vi "UHR-Fleezers Control (host) - 11.8.vi"() -> ()   [LabVIEW 2014] (continued)
                                tunnel: w980 -> [w981]
                                frame #0 {
                                n672 = property on="Trap Pos FB SP" class="DigNum (strict)"("Val(Sgnl)"=w981) -> ()  [unwired: 2 in, 2 out]
                                }
                                frame #1 {
                                n673 = Wait (ms)(milliseconds to wait=u32 700) -> ()  [unwired: 1 out]
                                }
                                frame #2 {
                                n674 = local read "Action (%)"() -> (w986:dbl)
                                n675 = Absolute Value(x=w986) -> (abs(x)=w985:dbl)
                                n676 = Greater?(x=w985, y=70.0) -> (0:w983:bool)
                                n677 = property on="Remove Action Offset" class="Bool (strict)"("Val(Sgnl)"=w983) -> ()  [unwired: 2 in, 2 out]
                                }
                                frame #3 {
                                n678 = for {
                                N: 4 -> [_]
                                n679 = flat-sequence {
                                frame #0 {
                                n680 = Wait (ms)(milliseconds to wait=u32 500) -> ()  [unwired: 1 out]
                                }
                                frame #1 {
                                n681 = local read "Action (%)"() -> (w992:dbl)
                                n682 = Absolute Value(x=w992) -> (abs(x)=w991:dbl)
                                n683 = Greater?(x=w991, y=70.0) -> (0:w989:bool)
                                n684 = property on="Remove Action Offset" class="Bool (strict)"("Val(Sgnl)"=w989) -> ()  [unwired: 2 in, 2 out]
                                }
                                }
                                }
                                }
                                frame #4 {
                                n685 = local read "Shift confocal"() -> (w996:bool)
                                n686 = local read "Mean"() -> (w999:dbl)
                                n687 = Greater?(x=w999, y=11.0) -> (0:w995:bool)
                                n688 = Not(x=w995) -> (.not. x?=w994:bool)
                                n689 = And(x=w994, y=w996) -> (x .and. y?=w993:bool)
                                n690 = And(x=w995, y=w996) -> (x .and. y?=w997:bool)
                                n691 = case shown="True" w997 {
                                frame False {
                                }
                                frame True {
                                n692 = local read "Confocal X 2 (V)"() -> (w1002:dbl)
                                n693 = local read "Confocal Y 2 (V)"() -> (w1003:dbl)
                                n694 = property on="AO2" class="Slide (strict)"("Val(Sgnl)"=w1002) -> ()  [unwired: 2 in, 2 out]
                                n695 = property on="AO1" class="Slide (strict)"("Val(Sgnl)"=w1003) -> ()  [unwired: 2 in, 2 out]
                                }
                                }
                                n696 = case shown="True" w993 {
                                frame False {
                                }
                                frame True {
                                n697 = local read "Confocal X 1 (V)"() -> (w1000:dbl)
                                n698 = local read "Confocal Y 1 (V)"() -> (w1001:dbl)
                                n699 = property on="AO1" class="Slide (strict)"("Val(Sgnl)"=w1001) -> ()  [unwired: 2 in, 2 out]
                                n700 = property on="AO2" class="Slide (strict)"("Val(Sgnl)"=w1000) -> ()  [unwired: 2 in, 2 out]
                                }
                                }
                                }
                                frame #5 {
                                n701 = Wait (ms)(milliseconds to wait=u32 1500) -> ()  [unwired: 1 out]
                                }
                                frame #6 {
                                n702 = property on="Remove Offset" class="Bool (strict)"("Val(Sgnl)"=TRUE ("Value (Signaling)")) -> ()  [unwired: 2 in, 2 out]
                                n703 = property on="Rem fb disp offset" class="Bool (strict)"("Val(Sgnl)"=TRUE ("Value (Signaling)")) -> ()  [unwired: 2 in, 2 out]
                                }
                                }
                                }
                                frame True {
                                n704 = flat-sequence {
                                tunnel: w1007 -> [w1008]
                                frame #0 {
                                n705 = property on="Trap D (MHz)" class="DigNum (strict)"("Val(Sgnl)"=w1008) -> ()  [unwired: 2 in, 2 out]
                                }
                                frame #1 {
                                n706 = Wait (ms)(milliseconds to wait=u32 500) -> ()  [unwired: 1 out]
                                }
                                frame #2 {
                                n707 = local read "Shift confocal"() -> (w1012:bool)
                                n708 = local read "Mean"() -> (w1010:dbl)
                                n709 = Greater?(x=w1010, y=11.0) -> (0:w1013:bool)
                                n710 = Not(x=w1013) -> (.not. x?=w1014:bool)
                                n711 = And(x=w1014, y=w1012) -> (x .and. y?=w1016:bool)
                                n712 = And(x=w1013, y=w1012) -> (x .and. y?=w1015:bool)
                                n713 = case shown="True" w1015 {
                                frame False {
                                }
                                frame True {
                                n714 = local read "Confocal Y 2 (V)"() -> (w1020:dbl)
                                n715 = local read "Confocal X 2 (V)"() -> (w1019:dbl)
                                n716 = property on="AO1" class="Slide (strict)"("Val(Sgnl)"=w1020) -> ()  [unwired: 2 in, 2 out]
                                n717 = property on="AO2" class="Slide (strict)"("Val(Sgnl)"=w1019) -> ()  [unwired: 2 in, 2 out]
                                }
                                }
                                n718 = case shown="True" w1016 {
                                frame False {
                                }
                                frame True {
                                n719 = local read "Confocal X 1 (V)"() -> (w1017:dbl)
                                n720 = local read "Confocal Y 1 (V)"() -> (w1018:dbl)
                                n721 = property on="AO2" class="Slide (strict)"("Val(Sgnl)"=w1017) -> ()  [unwired: 2 in, 2 out]
                                n722 = property on="AO1" class="Slide (strict)"("Val(Sgnl)"=w1018) -> ()  [unwired: 2 in, 2 out]
                                }
                                }
                                }
                                }
                                }
                                }
                                }
                              }
                            }
                            frame "Raster" {
                              n723 = property on="Trap Raster Scan" class="Bool (strict)"("Val(Sgnl)"=TRUE ("Value (Signaling)")) -> ()  [unwired: 2 in, 2 out]
                            }
                          }
                          n724 = local read "Time (s)"() -> (w953:dbl)
                          "Fl. High" <- TRUE ("Yanking")
                        }
                        frame #1 {
                          n725 = local read "Auto F Reset"() -> (w1022:bool)
                          n726 = case shown="True" w1022 {
                            tunnel: w1027 -> [_ w1031]
                            tunnel: w1026 -> [_ w1030]
                            tunnel: w1025 -> [_ w1029]
                            tunnel: w1023 -> [_ w1028]
                            frame False {
                            }
                            frame True {
                              n727 = node-c288() -> (w1033:T21)  [unwired: 4 out]
                              n728 = timed-loop {
                                timing: w1033 -> [_]
                                timing-out: [_] -> w1032
                                tunnel: w1031 -> [w1051]
                                tunnel: w1030 -> [w1050]
                                tunnel: w1029 -> [w1049]
                                tunnel: w1028 -> [w1048]
                                stop <- w1034 stop-if-true
                                n729 = node-c288() -> ()  [unwired: 2 out]
                                n730 = local read "Fl. D Thresh. (kHz)"() -> (w1042:dbl)
                                n731 = local read "Fl. Triggered..."() -> (w1047:bool)
                                n732 = local read "Delta Fl. 1"() -> (w1038:dbl)
                                n733 = local read "Delta Fl. 2"() -> (w1036:dbl)
                                n734 = local read "Stop All"() -> (w1045:bool)
                                n735 = local read "APD to Watch"() -> (w1037:bool)
                                n736 = Select(t=w1038, s=w1037, f=w1036) -> (s? t:f=w1035:dbl)
                                n737 = Not(x=w1047) -> (.not. x?=w1046:bool)
                                n738 = Multiply(x=w1042, y=1000.0) -> (x*y=w1041:dbl)
                                n739 = Negate(x=w1041) -> (-x=w1040:dbl)
                                n740 = Less?(x=w1035, y=w1040) -> (x < y?=w1044:bool)
                                n741 = Compound Arithmetic op=OR(w1044, w1045, w1046, "Reset Force") -> (w1034:bool)
                                n742 = case shown="True" w1034 {
                                tunnel: w1051 -> [_ w1066]
                                tunnel: w1050 -> [_ w1065]
                                tunnel: w1049 -> [_ w1055]
                                tunnel: w1048 -> [_ w1057]
                                frame False {
                                }
                                frame True {
                                n743 = local read "Time (s)"() -> (w1056:dbl)
                                n744 = case shown="\"Yank\"" w1065 {
                                tunnel: w1066 -> [_ w1069]
                                tunnel: w1057 -> [_ w1067]
                                frame "Image", Default {
                                }
                                frame "Yank" {
                                n745 = flat-sequence {
                                tunnel: [w1075] -> w1070
                                tunnel: w1069 -> [w1075]
                                tunnel: [w1071] -> w1068
                                tunnel: w1067 -> [w1071]
                                tunnel: w1070 -> [w1078]
                                tunnel: w1068 -> [w1076]
                                frame #0 {
                                n746 = local read "Yank Delay (s)"() -> (w1074:dbl)
                                n747 = Multiply(x=w1074, y=1000.0) -> (x*y=w1072:dbl)
                                n748 = Wait (ms)(milliseconds to wait=w1072) -> ()  [unwired: 1 out]
                                }
                                frame #1 {
                                n749 = local read "Yank to which?"() -> (w1077:bool)
                                n750 = case shown="False" w1077 {
                                tunnel: w1078 -> [_ w1106]
                                tunnel: w1076 -> [w1079 _]
                                frame False {
                                n751 = flat-sequence {
                                tunnel: w1079 -> [w1080]
                                frame #0 {
                                n752 = property on="Trap Pos FB SP" class="DigNum (strict)"("Val(Sgnl)"=w1080) -> ()  [unwired: 2 in, 2 out]
                                }
                                frame #1 {
                                n753 = Wait (ms)(milliseconds to wait=u32 700) -> ()  [unwired: 1 out]
                                }
                                frame #2 {
                                n754 = local read "Action (%)"() -> (w1085:dbl)
                                n755 = Absolute Value(x=w1085) -> (abs(x)=w1084:dbl)
                                n756 = Greater?(x=w1084, y=70.0) -> (0:w1082:bool)
                                n757 = property on="Remove Action Offset" class="Bool (strict)"("Val(Sgnl)"=w1082) -> ()  [unwired: 2 in, 2 out]
                                }
                                frame #3 {
                                n758 = for {
                                N: 4 -> [_]
                                n759 = flat-sequence {
                                frame #0 {
                                n760 = Wait (ms)(milliseconds to wait=u32 500) -> ()  [unwired: 1 out]
                                }
                                frame #1 {
                                n761 = local read "Action (%)"() -> (w1091:dbl)
                                n762 = Absolute Value(x=w1091) -> (abs(x)=w1090:dbl)
                                n763 = Greater?(x=w1090, y=70.0) -> (0:w1088:bool)
                                n764 = property on="Remove Action Offset" class="Bool (strict)"("Val(Sgnl)"=w1088) -> ()  [unwired: 2 in, 2 out]
                                }
                                }
                                }
                                }
                                frame #4 {
                                n765 = local read "Shift confocal"() -> (w1096:bool)
                                n766 = local read "Mean"() -> (w1098:dbl)
                                n767 = Greater?(x=w1098, y=11.0) -> (0:w1095:bool)
                                n768 = Not(x=w1095) -> (.not. x?=w1094:bool)
                                n769 = And(x=w1095, y=w1096) -> (x .and. y?=w1093:bool)
                                n770 = And(x=w1094, y=w1096) -> (x .and. y?=w1092:bool)
                                n771 = case shown="True" w1093 {
                                frame False {
                                }
                                frame True {
                                n772 = local read "Confocal Y 2 (V)"() -> (w1102:dbl)
                                n773 = local read "Confocal X 2 (V)"() -> (w1101:dbl)
                                n774 = property on="AO2" class="Slide (strict)"("Val(Sgnl)"=w1101) -> ()  [unwired: 2 in, 2 out]
                                n775 = property on="AO1" class="Slide (strict)"("Val(Sgnl)"=w1102) -> ()  [unwired: 2 in, 2 out]
                                }
                                }
                                n776 = case shown="True" w1092 {
                                frame False {
                                }
                                frame True {
                                n777 = local read "Confocal X 1 (V)"() -> (w1099:dbl)
                                n778 = local read "Confocal Y 1 (V)"() -> (w1100:dbl)
                                n779 = property on="AO1" class="Slide (strict)"("Val(Sgnl)"=w1100) -> ()  [unwired: 2 in, 2 out]
                                n780 = property on="AO2" class="Slide (strict)"("Val(Sgnl)"=w1099) -> ()  [unwired: 2 in, 2 out]
                                }
                                }
                                }
                                frame #5 {
                                n781 = Wait (ms)(milliseconds to wait=u32 1500) -> ()  [unwired: 1 out]
                                }
                                frame #6 {
                                n782 = property on="Rem fb disp offset" class="Bool (strict)"("Val(Sgnl)"=TRUE ("Value (Signaling)")) -> ()  [unwired: 2 in, 2 out]
                                n783 = property on="Remove Offset" class="Bool (strict)"("Val(Sgnl)"=TRUE ("Value (Signaling)")) -> ()  [unwired: 2 in, 2 out]
                                }
                                }
                                }
                                frame True {
                                n784 = flat-sequence {
                                tunnel: w1106 -> [w1107]
                                frame #0 {
                                n785 = property on="Trap D (MHz)" class="DigNum (strict)"("Val(Sgnl)"=w1107) -> ()  [unwired: 2 in, 2 out]
                                }
                                frame #1 {
                                n786 = Wait (ms)(milliseconds to wait=u32 500) -> ()  [unwired: 1 out]
                                }
                                frame #2 {
                                n787 = local read "Shift confocal"() -> (w1113:bool)
                                n788 = local read "Mean"() -> (w1115:dbl)
                                n789 = Greater?(x=w1115, y=11.0) -> (0:w1112:bool)
                                n790 = Not(x=w1112) -> (.not. x?=w1111:bool)
                                n791 = And(x=w1112, y=w1113) -> (x .and. y?=w1110:bool)
                                n792 = And(x=w1111, y=w1113) -> (x .and. y?=w1109:bool)
                                n793 = case shown="True" w1110 {
                                frame False {
                                }
                                frame True {
                                n794 = local read "Confocal Y 2 (V)"() -> (w1119:dbl)
                                n795 = local read "Confocal X 2 (V)"() -> (w1118:dbl)
                                n796 = property on="AO2" class="Slide (strict)"("Val(Sgnl)"=w1118) -> ()  [unwired: 2 in, 2 out]
                                n797 = property on="AO1" class="Slide (strict)"("Val(Sgnl)"=w1119) -> ()  [unwired: 2 in, 2 out]
                                }
                                }
                                n798 = case shown="True" w1109 {
                                frame False {
                                }
                                frame True {
                                n799 = local read "Confocal Y 1 (V)"() -> (w1117:dbl)
                                n800 = local read "Confocal X 1 (V)"() -> (w1116:dbl)
                                n801 = property on="AO2" class="Slide (strict)"("Val(Sgnl)"=w1116) -> ()  [unwired: 2 in, 2 out]
                                n802 = property on="AO1" class="Slide (strict)"("Val(Sgnl)"=w1117) -> ()  [unwired: 2 in, 2 out]
                                }
                                }
                                }
                                }
                                }
                                }
                                }
                                }
                                }
                                }
                                n803 = local read "Messages"() -> (w1064:string)
                                n804 = Subtract(x=w1056, y=w1055) -> (x-y=w1062:dbl)
                                "Duration (s)" <- w1062
                                n805 = Number To Decimal String(number=w1062, width (-)=i16 0) -> (decimal integer string=w1060:string)
                                n806 = Concatenate Strings(w1060, " s fluorescence event." ("string")) -> (w1058:string)
                                n807 = call "Update messages.vi"("Message to add"=w1058, "Old message string"=w1064) -> ("New message string"=w1063:string)
                                n808 = local write "Reset Force"(FALSE ("Reset Force")) -> ()
                                n809 = local write "Waiting"(TRUE ("Waiting")) -> ()
                                n810 = local write "Messages"(w1063) -> ()
                                n811 = local write "Fl. High"(FALSE ("Fl. High")) -> ()
                                n812 = call <vilib>:"Beep.vi"() -> ()  [unwired: 3 in, 9 out]
                                }
                                }
                                n813 = node-c288() -> ()  [unwired: 2 out]
                              }
                              n814 = node-c288(w1032) -> ()  [unwired: 1 out]
                            }
                          }
                        }
                      }
                      n815 = local read "Trap Pos FB SP"() -> (w940:fxp<+/-,16,1>)
                      n816 = local read "Trap D (MHz)"() -> (w945:dbl)
                    }
                  }
                }
                frame #1 {
                  n817 = local read "Stop All"() -> (w1129:bool)
                  n818 = local read "Fl. Triggered..."() -> (w1127:bool)
                  n819 = Not(x=w1127) -> (.not. x?=w1128:bool)
                  n820 = Or(x=w1128, y=w1129) -> (x .or. y?=w1126:bool)
                }
              }
              n821 = case shown="True" w715 {
                frame False {
                }
                frame True {
                  n822 = local read "Confocal Y 1 (V)"() -> (w725:dbl)
                  n823 = local read "Confocal X 1 (V)"() -> (w724:dbl)
                  n824 = property on="AO2" class="Slide (strict)"("Val(Sgnl)"=w724) -> ()  [unwired: 2 in, 2 out]
                  n825 = property on="AO1" class="Slide (strict)"("Val(Sgnl)"=w725) -> ()  [unwired: 2 in, 2 out]
                }
              }
              n826 = case shown="True" w715 {
                frame False {
                }
                frame True {
                  w723 = FALSE ("Fl. High")
                  n827 = local write "Waiting"(w723) -> ()
                  n828 = local write "Fl. High"(w723) -> ()
                }
              }
              n829 = node-c288() -> ()  [unwired: 2 out]
            }
            n830 = node-c288(w713) -> ()  [unwired: 1 out]
          }
        }
      }
      event "Stop All": Value Change {
        n831 = event-data() -> ()  [unwired: 7 out]
        n832 = local read "Stop All"() -> (w1134:bool)
      }
    }
    n833 = node-c288() -> ()  [unwired: 2 out]
  }
  n834 = property on="Saved trap pos" class="WFGraph (strict)"("Visible"=TRUE) -> ()  [unwired: 2 in, 2 out]
  n835 = property on="Trap Delta Graph" class="WFGraph (strict)"("Visible"=FALSE) -> ()  [unwired: 2 in, 2 out]
  n836 = local write "Trap pos"(TRUE ("Trap pos")) -> ()
  n837 = node-c288(2 ("Processor")) -> (w108:T21)  [unwired: 3 out]
  n838 = timed-loop "Control parameters (event loop)" {
    tunnel: w18 -> [w1143]
    shift-right: [w1142] -> _
    shift-left: errorcluster {"status"=FALSE, "code"=0, "source"=""} ("error out") -> [w1141]
    tunnel: [w1140] -> _
    timing: w108 -> [_]
    timing-out: [_] -> w107
    tunnel: w81 -> [w1139]
    tunnel: w22 -> [w1138]
    tunnel: w21 -> [w1137]
    tunnel: w20 -> [w1136]
    tunnel: w19 -> [w1135]
    stop <- w1140 stop-if-true
    n839 = node-c288() -> ()  [unwired: 2 out]
    n840 = event shown="[46] \"Sample Channel Flow\": Value Change" {
      selector: _ -> [_ _ _ _ _ _ _ _ _ _ _ _ _ _ _ _ _ _ _ _ _ _ _ _ _ _ _ _ _ _ _ _ _ _ _ _ _ _ _ _ _ _ _ _ _ _ _ _ _ _ _ _ _ _ _ _ _ _ _ _ _ _ _ _ _ _ _ _ _ _ _ _ _ _ _ _ _ _ _ _]
      dyn-events: _ -> [_ _ _ _ _ _ _ _ _ _ _ _ _ _ _ _ _ _ _ _ _ _ _ _ _ _ _ _ _ _ _ _ _ _ _ _ _ _ _ _ _ _ _ _ _ _ _ _ _ _ _ _ _ _ _ _ _ _ _ _ _ _ _ _ _ _ _ _ _ _ _ _ _ _ _ _ _ _ _ _]
      timeout: _ -> [_ _ _ _ _ _ _ _ _ _ _ _ _ _ _ _ _ _ _ _ _ _ _ _ _ _ _ _ _ _ _ _ _ _ _ _ _ _ _ _ _ _ _ _ _ _ _ _ _ _ _ _ _ _ _ _ _ _ _ _ _ _ _ _ _ _ _ _ _ _ _ _ _ _ _ _ _ _ _ _]
      tunnel: w1143 -> [w1181 _ _ _ w1219 _ w1241 _ _ _ _ w1307 _ _ w1350 w1356 w1361 w1367 w1403 w1421 w1428 _ w1440 w1444 w1455 w1466 w1477 w1488 w1499 w1510 w1537 w1631 w1638 w1676 _ _ w1736 w1740 w1751 w1755 w1759 _ w1767 _ _ _ _ _ _ _ _ _ _ _ _ _ _ _ _ _ w2148 _ w2165 _ w2172 w2190 _ w2197 w2205 w2220 w2231 w2237 _ w2246 _ w2265 _ _ _ w2340]
      tunnel: [w1180 _ _ _ w1209 _ w1240 _ _ w1272 _ w1286 _ _ w1349 w1352 w1358 w1364 w1402 w1419 w1427 _ w1438 _ w1449 w1460 w1471 w1482 w1493 w1504 w1535 w1629 w1636 w1674 _ _ w1734 w1738 w1741 w1753 w1757 _ w1765 _ _ _ _ _ _ _ _ _ _ _ _ _ _ _ _ _ w2146 _ _ _ _ w2187 _ _ _ _ _ _ _ _ _ _ _ _ _ w2338] -> w1142
      tunnel: w1141 -> [w1179 _ _ _ w1218 _ w1239 _ _ w1272 _ w1306 _ _ w1348 w1351 w1357 w1363 w1401 w1420 w1426 _ w1439 w1443 w1454 w1465 w1476 w1487 w1498 w1509 w1536 w1630 w1637 w1675 _ _ w1735 w1739 w1750 w1754 w1758 _ w1766 _ _ _ _ _ _ _ _ _ _ _ _ _ _ _ _ _ w2147 _ w2164 _ w2171 w2189 _ w2196 w2204 w2219 w2230 w2236 _ w2245 _ w2264 _ _ _ w2339]
      tunnel: [_ _ _ _ _ _ _ _ _ w1271 _ _ _ _ _ _ _ _ _ _ _ _ _ _ _ _ _ _ _ _ _ _ _ _ _ _ _ _ _ _ _ _ _ _ _ _ _ _ _ _ _ _ _ _ _ _ _ _ _ _ _ _ _ _ _ _ _ _ _ _ _ _ _ _ _ _ _ _ _ _] -> w1140
      tunnel: [_ _ _ _ _ _ _ "Round T1 X" _ _ _ _ _ _ _ _ _ _ _ _ _ _ _ _ _ _ _ _ _ _ _ _ _ _ _ _ _ _ _ _ _ _ _ _ _ _ _ _ _ _ _ _ _ _ _ _ _ _ _ _ _ _ _ _ _ _ _ _ _ _ _ _ _ _ _ _ _ _ _ _] -> _
      tunnel: [_ _ _ "Adjust Scale\nto Mean" _ _ _ _ _ _ _ _ _ _ _ _ _ _ _ _ _ _ "Test ttrig" _ _ _ _ _ _ _ _ _ _ _ _ _ _ _ _ _ _ _ _ _ _ _ _ _ _ _ "Flush Sample" "Flush Pump 3" "Flush Pump 1" "Clear Volume" _ _ _ _ _ _ _ _ _ _ _ _ _ _ _ _ _ _ _ _ _ _ _ _ _ _] -> _
      tunnel: [_ _ _ _ _ _ _ _ "Round T2 X" _ "Delayed Interlace Start" _ _ _ _ _ _ _ _ _ _ _ _ _ _ _ _ _ _ _ _ _ _ _ _ _ _ _ _ _ _ _ _ _ _ _ _ _ _ _ _ _ _ _ _ _ _ _ _ _ _ _ _ _ _ _ _ _ _ _ _ _ _ _ _ _ _ _ _ _] -> _
      tunnel: w1139 -> [_ _ _ _ _ _ _ _ _ _ _ _ _ _ _ _ _ _ _ _ _ _ _ _ _ _ _ _ _ _ _ _ _ _ _ _ _ _ _ _ _ _ _ _ _ _ w1925 w1943 w1950 w1955 w1961 _ _ w2060 _ _ _ _ _ _ _ _ _ _ _ _ _ _ _ _ _ _ _ _ _ _ _ _ _ _]
      tunnel: w1138 -> [_ _ _ _ _ _ _ _ _ _ _ _ _ _ _ _ _ _ _ _ _ _ _ _ _ _ _ _ _ _ _ _ _ _ _ _ _ _ _ _ _ _ _ _ w1841 _ _ _ _ _ _ w1991 _ _ w2067 _ w2076 _ w2090 _ _ _ _ _ _ _ _ _ _ _ _ _ _ _ _ _ _ _ _ _]
      tunnel: w1137 -> [_ _ _ _ _ _ _ _ _ _ _ _ _ _ _ _ _ _ _ _ _ _ _ _ _ _ _ _ _ _ _ _ _ _ _ _ _ _ _ _ _ _ _ _ _ _ _ _ _ _ _ _ _ _ _ _ _ _ _ _ _ _ _ _ _ _ _ _ _ _ _ _ _ _ _ _ _ _ _ _]
      tunnel: w1136 -> [_ _ _ _ _ _ _ _ _ _ _ _ _ _ _ _ _ _ _ _ _ _ _ _ _ _ _ _ _ _ _ _ _ _ _ _ _ _ _ _ _ _ _ w1778 _ _ _ _ _ _ _ _ w2021 _ _ w2072 _ w2083 _ w2115 _ _ _ _ _ _ _ _ _ _ _ _ _ _ _ _ _ _ _ _]
      tunnel: w1135 -> [_ _ _ _ _ _ _ _ _ _ _ _ _ _ _ _ _ _ _ _ _ _ _ _ _ _ _ _ _ _ _ _ _ _ _ _ _ _ _ _ _ _ _ _ _ _ _ _ _ _ _ _ _ _ _ _ _ _ _ _ _ _ _ _ _ _ _ _ _ _ _ _ _ _ _ _ _ _ _ _]
      event "AI Count (ticks)", "Sets to FIFO (Traps)", "Save ave N", "FPGA Ave.", "# Samples/channel", "N sets to save": Value Change {
        # "So that if 'Save ave N' is updated, the AOD scanning code updates too."
        n841 = event-data() -> ()  [unwired: 6 out]
        n842 = local read "AI Count (ticks)"() -> (w1161:u32)
        n843 = Boolean To (0,1)(Boolean="Sets to FIFO (Traps)") -> (0, 1=w1171:cluster{"Set 1":i16, "Set 2":i16, "Set 3":i16})
        n844 = Cluster To Array(cluster=w1171) -> (array=w1170:i16[])
        n845 = xnode "Read/Write Control"("FPGA VI Reference In"=w1181, "error in"=w1179, "ai count"=w1161, "AI1 Sets to FIFO"="Sets to FIFO (Traps)", "N of AI1 Int Acq Sets"="N Acq Sets (Traps + Fl.)") -> ("error out"=w1180:errorcluster)  [unwired: 1 out]
        n846 = To Unsigned Long Integer(number=w1170) -> (unsigned 32bit integer=w1150:u32[])
        n847 = local read "Scan steps (AOD)"() -> (w1172:u64)
        n848 = Multiply(x=w1161, y="N Acq Sets (Traps + Fl.)") -> (x*y=w1159:u32)
        n849 = Divide(x=40000000.0, y=w1161) -> (x/y=w1153:dbl)
        "AI rate (Hz)" <- w1153
        "Ave. Rate (Hz)" <- w1153
        n850 = Add Array Elements(numeric array=w1150) -> (sum=w1162:u32)
        "Trap Sets" <- w1162
        n851 = Reciprocal(x=w1153) -> (1/x=→"Ave. Period (s)":dbl)
        n852 = property on="Scan steps (AOD)" class="DigNum (strict)"("Val(Sgnl)"=w1172) -> ()  [unwired: 2 in, 2 out]
        n853 = Divide(x=w1153, y="N Acq Sets (Traps + Fl.)") -> (x/y=w1176:dbl)
        "Data Rate (Hz)" <- w1176
        n854 = Reciprocal(x=w1176) -> (1/x=→"Data Period (s)":dbl)
        n855 = local read "Save ave N"() -> (w1175:dbl)
        n856 = Divide(x=w1176, y=w1175) -> (x/y=w1174:dbl)
        "Save Data Rate (Hz)" <- w1174
        n857 = Reciprocal(x=w1174) -> (1/x=→"Save Data Period (s)":dbl)
        n858 = Multiply(x=w1159, y="# Samples/trap") -> (x*y=w1157:u32)
        "Counts/DMA" <- w1157
        n859 = property on="Trap Disp. Downsample" class="DigNum (strict)"("Maximum"="# Samples/trap") -> ()  [unwired: 2 in, 2 out]
        n860 = Multiply(x=w1162, y="# Samples/trap") -> (x*y=w1151:u32)
        "# Samples/channel" <- w1151
        n861 = Multiply(x=w1151, y=u32 8) -> (x*y=→"Trap AI Elements/DMA read":u32)
        n862 = local read "APD Int. Count"() -> (w1158:u32)
        n863 = Multiply(x=w1151, y=u32 3) -> (x*y=→"Trap Pos Elements/DMA read":u32)
        n864 = Divide(x=w1157, y=w1158) -> (x/y=w1148:dbl)
        "APD Samples/FIFO Acq." <- w1148
        n865 = Divide(x=w1157, y=40000000.0) -> (x/y=w1155:dbl)
        "DMA Update Period (s)" <- w1155
        n866 = Multiply(x=2.0, y=w1148) -> (x*y=→"APD Elements/DMA read":dbl)
        n867 = property on="APD Disp. Downsample" class="DigNum (strict)"("Maximum"=w1148) -> ()  [unwired: 2 in, 2 out]
        n868 = local read "N sets to save"() -> (w1168:u32)
        n869 = Multiply(x=w1155, y=w1168) -> (x*y=→"Total Time (s)":dbl)
        "FPGA Averaging" <- FALSE ("FPGA Averaging")
      }
      event "Remove Offset": Value Change {
        n870 = event-data() -> ()  [unwired: 7 out]
        n871 = local write "Remove Offset"(FALSE ("Remove Offset")) -> ()
        n872 = local read "Bead Mean (nm)"() -> (w1183:dbl)
        n873 = local read "Offset (nm)"() -> (w1184:dbl)
        n874 = Add(x=w1183, y=w1184) -> (x+y=w1182:dbl)
        n875 = local write "Offset (nm)"(w1182) -> ()
        n876 = disable-structure shown="Disabled" {
          frame Disabled {
            n877 = local read "Bead Mean (nm)"() -> (w1189:dbl)
            n878 = Add(y=w1189) -> (x=w1188:dbl, x+y=w1187:dbl)
            n879 = Subtract(x=w1189, y=w1188) -> (x-y=w1186:dbl)
            n880 = property on="Bead Separation" class="WFChart (strict)"("YScale.Minimum"=w1186) -> ()  [unwired: 2 in, 2 out]
            n881 = property on="Bead Separation" class="WFChart (strict)"("YScale.Maximum"=w1187) -> ()  [unwired: 2 in, 2 out]
          }
          frame Enabled {
          }
        }
      }
      event "Detector Type": Value Change {
        n882 = event-data() -> ()  [unwired: 7 out]
        n883 = local read "AI labels"() -> (w1190:string[])
        n884 = property on="High Res. Display" class="Ring (strict)"("Strings []"=w1190) -> ()  [unwired: 2 in, 2 out]
        n885 = Build Array (concatenate)(w1190, "none") -> (w1191:string[])
        n886 = property on="FFT 1 Choice 1" class="Ring (strict)"("Strings []"=w1191) -> ()  [unwired: 2 in, 2 out]
        n887 = property on="FFT 1 Choice 2" class="Ring (strict)"("Strings []"=w1191) -> ()  [unwired: 2 in, 2 out]
        n888 = property on="FFT 2 Choice 1" class="Ring (strict)"("Strings []"=w1191) -> ()  [unwired: 2 in, 2 out]
        n889 = property on="FFT 2 Choice 2" class="Ring (strict)"("Strings []"=w1191) -> ()  [unwired: 2 in, 2 out]
        n890 = Bundle("APD 1", "APD 2") -> (w1194:cluster{string, string})  [unwired: 1 out]
        n891 = Cluster To Array(cluster=w1194) -> (array=w1192:string[])
        n892 = Build Array (concatenate)(w1192, w1191) -> (w1196:string[])
        n893 = Array Size(array=w1196) -> (size(s)=w1197:i32)
        n894 = property on="Signals to Plot" class="LstBox (strict)"("Item Names"=w1196) -> ()  [unwired: 2 in, 2 out]
        n895 = property on="Signals to Plot" class="LstBox (strict)"("Number of Rows"=w1197) -> ()  [unwired: 2 in, 2 out]
        n896 = property on="All Signals" class="WFChart (strict)"("LegNumRows"=w1197) -> ()  [unwired: 2 in, 2 out]
      }
      event "Adjust Scale\nto Mean": Value Change {
        n897 = event-data() -> ()  [unwired: 7 out]
        n898 = local read "APD 1 Rate (Hz)"() -> (w1206:dbl)
        n899 = Multiply(x=1000.0, y="Above (kHz)") -> (x*y=w1204:dbl)
        n900 = Multiply(x=1000.0, y="Below (kHz)") -> (x*y=w1202:dbl)
        n901 = Add(x=w1204, y=w1206) -> (x+y=w1199:dbl)
        n902 = Subtract(x=w1206, y=w1202) -> (x-y=w1200:dbl)
        n903 = property on="APD Chart" class="WFChart (strict)"("YScale.Minimum"=w1200) -> ()  [unwired: 2 in, 2 out]
        n904 = property on="APD Chart" class="WFChart (strict)"("YScale.Maximum"=w1199) -> ()  [unwired: 2 in, 2 out]
      }
      event "Phase adj. (AI1)", "+ phase (AI1)", "- phase (AI1)": Value Change {
        n905 = event-data() -> ()  [unwired: 7 out]
        n906 = Negate(x="Phase adj. (AI1)") -> (-x=w1216:i16)
        n907 = Select(t=w1216, s="- phase (AI1)", f="Phase adj. (AI1)") -> (s? t:f=w1215:i16)
        n908 = xnode "Read/Write Control"("FPGA VI Reference In"=w1219, "error in"=w1218, "Phase count adjustment"=w1215) -> ("FPGA VI Reference Out"=w1214:T19, "error out"=w1213:errorcluster)
        n909 = Or(x="- phase (AI1)", y="+ phase (AI1)") -> (x .or. y?=w1210:bool)
        n910 = xnode "Read/Write Control"("FPGA VI Reference In"=w1214, "error in"=w1213, "+ phase"=w1210) -> ("error out"=w1209:errorcluster)  [unwired: 1 out]
      }
      event "Signals to Plot": Double Click {
        w1222 = u32 9868950 ("Color Box")
        n911 = event-data() -> ("Row"=w1224:i32)  [unwired: 9 out]
        n912 = property on="All Signals" class="WFChart (strict)"("Active Plot"=w1224) -> (error out=w1235:errorcluster)  [unwired: 2 in, 1 out]
        n913 = property on="All Signals" class="WFChart (strict)" props=["Plot", "Visible?", "Plot", "Plot Color"](error in=w1235) -> (error out=w1234:errorcluster, "Plot.Visible?"=w1233:bool)  [unwired: 1 in, 2 out]
        n914 = Select(t=FALSE ("Plot.Visible"), s=w1233, f=TRUE ("Plot.Visible")) -> (s? t:f=w1228:bool)
        n915 = property on="All Signals" class="WFChart (strict)"(error in=w1234, "Plot.Visible?"=w1228) -> (error out=w1230:errorcluster)  [unwired: 1 in, 1 out]
        n916 = property on="All Signals" class="WFChart (strict)"(error in=w1230) -> (error out=w1225:errorcluster, "Plot.Plot Color"=w1229:u32)  [unwired: 1 in, 1 out]
        n917 = property on="Signals to Plot" class="LstBox (strict)"(error in=w1225, "Active Row"=w1224) -> (error out=w1223:errorcluster)  [unwired: 1 in, 1 out]
        n918 = Select(t=w1229, s=w1228, f=u32 0) -> (s? t:f=w1226:u32)
        n919 = property on="Signals to Plot" class="LstBox (strict)"(error in=w1223, "CellFontColor"=w1226, "SelColor"=w1222, "CellBG"=w1222, "CellFontSize"=u32 20 ("Active Row:Cell Font:Size"), "CellFontBold"=TRUE ("Active Row:Cell Font:Bold")) -> ()  [unwired: 1 in, 2 out]
      }
      event "BD 1 Frequency 1 (MHz)", "BD 1 Frequency 2 (MHz)", "BD 1 Frequency 3 (MHz)", "BD 2 Frequency 1 (MHz)", "BD 2 Frequency 2 (MHz)", "BD 2 Frequency 3 (MHz)", "Trap D (MHz)": Value Change {
        n920 = event-data() -> ("CtlRef"=w1238:refnum<vi>)  [unwired: 6 out]
        n921 = control-ref of="Trap D (MHz)"() -> (w1237:refnum<vi>)
        n922 = Equal?(x=w1237, y=w1238) -> (x = y?=w1236:bool)
        n923 = case shown="False" "Oscillate Set 1" {
          tunnel: w1241 -> [w1261 _]
          tunnel: [w1260 w1264] -> w1240
          tunnel: w1239 -> [w1259 w1264]
          tunnel: w1236 -> [w1244 _]
          frame False {
            n924 = local read "BD 1 Frequency 2 (MHz)"() -> (w1248:dbl)
            n925 = local read "BD 1 Frequency 1 (MHz)"() -> (w1246:dbl)
            n926 = Subtract(x=w1248, y="Trap D (MHz)") -> (x-y=w1245:dbl)
            n927 = Select(t=w1245, s=w1244, f=w1246) -> (s? t:f=w1243:dbl)
            n928 = local read "Y RF Frequency Limits (MHz)"() -> (w1249:T16)
            n929 = local read "X RF Frequency Limits (MHz)"() -> (w1250:T16)
            n930 = local read "BD 1 Frequency 3 (MHz)"() -> (w1262:dbl)
            n931 = local write "BD 1 Frequency 1 (MHz)"(w1243) -> ()
            n932 = local read "BD 2 Frequency 1 (MHz)"() -> (w1253:dbl)
            n933 = local read "BD 2 Frequency 2 (MHz)"() -> (w1252:dbl)
            n934 = local read "BD 2 Frequency 3 (MHz)"() -> (w1263:dbl)
            n935 = call "set RF board frequency - interlace.vi"("Board 2 Frequency Limits"=w1249, "Board 1 Frequency Limits"=w1250, "error in"=w1259, "FPGA VI Reference In"=w1261, "Board 2 Frequency 3 (MHz)"=w1263, "Board 1 Frequency 3 (MHz)"=w1262, "Board 2 Frequency 2 (MHz)"=w1252, "Board 2 Frequency 1 (MHz)"=w1253, "Board 1 Frequency 2 (MHz)"=w1248, "Board 1 Frequency 1  (MHz)"=w1243) -> ("error out"=w1260:errorcluster)  [unwired: 1 out]
            n936 = Subtract(x=w1253, y=w1252) -> (x-y=w1257:dbl)
            n937 = Subtract(x=w1243, y=w1248) -> (x-y=w1258:dbl)
            n938 = Square(x=w1257) -> (x^2=w1255:dbl)
            n939 = Square(x=w1258) -> (x^2=w1256:dbl)
            n940 = Add(x=w1256, y=w1255) -> (x+y=w1254:dbl)
            n941 = Square Root(x=w1254) -> (sqrt(x)=w1251:dbl)
            n942 = local write "Trap D (MHz)"(w1251) -> ()
            n943 = property on="Initial D (MHz)" class="DigNum (strict)"("Val(Sgnl)"=w1251) -> ()  [unwired: 2 in, 2 out]
          }
          frame True {
          }
        }
      }
      event "Round T1 X": Value Change {
        n944 = event-data() -> ()  [unwired: 7 out]
        n945 = local read "BD 1 Frequency 1 (MHz)"() -> (w1267:dbl)
        n946 = Round To Nearest(number=w1267) -> (nearest integer value=w1266:dbl)
        n947 = property on="BD 1 Frequency 1 (MHz)" class="DigNum (strict)"("Val(Sgnl)"=w1266) -> ()  [unwired: 2 in, 2 out]
      }
      event "Round T2 X": Value Change {
        n948 = event-data() -> ()  [unwired: 7 out]
        n949 = local read "BD 1 Frequency 2 (MHz)"() -> (w1269:dbl)
        n950 = Round To Nearest(number=w1269) -> (nearest integer value=w1268:dbl)
        n951 = property on="BD 1 Frequency 2 (MHz)" class="DigNum (strict)"("Val(Sgnl)"=w1268) -> ()  [unwired: 2 in, 2 out]
      }
      event "Stop All": Value Change {
        n952 = event-data() -> ()  [unwired: 7 out]
        n953 = local read "Stop All"() -> (w1271:bool)
      }
      event "Delayed Interlace Start": Value Change {
        n954 = event-data() -> ()  [unwired: 7 out]
        n955 = flat-sequence {
          frame #0 {
            n956 = Multiply(x="Delay to Interlace (s)", y=1000.0) -> (x*y=w1274:dbl)
            n957 = Wait (ms)(milliseconds to wait=w1274) -> ()  [unwired: 1 out]
          }
          frame #1 {
            n958 = property on="Green laser mode" class="RadioBtnsControl (strict)"("Val(Sgnl)"=enum32{"Laser ON", "Laser OFF", "Interlace"}."Interlace" ("Value (Signaling)")) -> ()  [unwired: 2 in, 2 out]
          }
        }
      }
      event "BD 1 Amplitude 1 (%)", "BD 1 Amplitude 2 (%)", "BD 1 Amplitude 3 (%)", "BD 2 Amplitude 1 (%)", "BD 2 Amplitude 2 (%)", "BD 2 Amplitude 3 (%)", "Trap 1 ON", "Trap 2 ON", "Trap 3 ON", "Feedback On/Off", "All FB On/Off": Value Change {
        w1298 = i16 1 ("f")
        n959 = event-data() -> ()  [unwired: 7 out]
        n960 = local write "Trap 1 (ON/OFF)"("Trap 1 ON") -> ()
        n961 = local write "Trap 2 (ON/OFF)"("Trap 2 ON") -> ()
        n962 = Boolean To (0,1)(Boolean="Trap 3 ON") -> (0, 1=w1299:i16)
        n963 = Boolean To (0,1)(Boolean="Trap 1 ON") -> (0, 1=w1300:i16)
        n964 = Boolean To (0,1)(Boolean="Trap 2 ON") -> (0, 1=w1301:i16)
        n965 = Select(t=w1301, s="Trap ON/OFF X or Y Amp?", f=w1298) -> (s? t:f=w1296:i16)
        n966 = Select(t=w1300, s="Trap ON/OFF X or Y Amp?", f=w1298) -> (s? t:f=w1297:i16)
        n967 = Select(t=w1299, s="Trap ON/OFF X or Y Amp?", f=w1298) -> (s? t:f=w1295:i16)
        n968 = Select(t=w1298, s="Trap ON/OFF X or Y Amp?", f=w1301) -> (s? t:f=w1293:i16)
        n969 = Select(t=w1298, s="Trap ON/OFF X or Y Amp?", f=w1300) -> (s? t:f=w1294:i16)
        n970 = Select(t=w1298, s="Trap ON/OFF X or Y Amp?", f=w1299) -> (s? t:f=w1292:i16)
        n971 = And(x="All FB On/Off", y="Feedback On/Off") -> (x .and. y?=w1290:cluster{"Set 1":bool, "Set 2":bool})
        n972 = local read "BD 1 Amplitude 1 (%)"() -> (w1310:dbl)
        n973 = local read "BD 1 Amplitude 2 (%)"() -> (w1309:dbl)
        n974 = local read "BD 1 Amplitude 3 (%)"() -> (w1308:dbl)
        n975 = Unbundle By Name(w1290) -> ("Set 1"=w1285:bool, "Set 2"=w1282:bool)
        n976 = local read "Y RF Amplitude Limits (%)"() -> (w1278:T16)
        n977 = local read "X RF Amplitude Limits (%)"() -> (w1279:T16)
        n978 = local read "BD 2 Amplitude 1 (%)"() -> (w1311:dbl)
        n979 = local read "BD 2 Amplitude 2 (%)"() -> (w1312:dbl)
        n980 = local read "BD 2 Amplitude 3 (%)"() -> (w1313:dbl)
        n981 = And(x="Trap 2 ON", y=w1282) -> (x .and. y?=w1280:bool)
        n982 = And(x="Trap 1 ON", y=w1285) -> (x .and. y?=w1283:bool)
        n983 = Multiply(x=w1297, y=w1310) -> (x*y=w1305:dbl)
        n984 = Multiply(x=w1309, y=w1296) -> (x*y=w1303:dbl)
        n985 = Multiply(x=w1308, y=w1295) -> (x*y=w1304:dbl)
        n986 = Multiply(x=w1311, y=w1294) -> (x*y=w1314:dbl)
        n987 = Multiply(x=w1312, y=w1293) -> (x*y=w1315:dbl)
        n988 = Multiply(x=w1313, y=w1292) -> (x*y=w1316:dbl)
        n989 = call "set RF board amplitude - interlace.vi"("Board 2 Amplitude Limits"=w1278, "Board 1 Amplitude Limits"=w1279, "error in"=w1306, "FPGA VI Reference In"=w1307, "Board 2 Amplitude 3 (%)"=w1316, "Board 1 Amplitude 3 (%)"=w1304, "Board 2 Amplitude 2 (%)"=w1315, "Board 2 Amplitude 1 (%)"=w1314, "Board 1 Amplitude 2 (%)"=w1303, "Board 1 Amplitude 1 (%)"=w1305) -> ("error out"=w1287:errorcluster, "FPGA VI Reference Out"=w1288:T19)
        n990 = xnode "Read/Write Control"("FPGA VI Reference In"=w1288, "error in"=w1287, "FB On/Off Set 1"=w1283, "FB On/Off Set 2"=w1280) -> ("error out"=w1286:errorcluster)  [unwired: 1 out]
      }
      event "Load parameters": Value Change {
        n991 = event-data() -> ()  [unwired: 7 out]
        n992 = property on="Saved AOD Raster Scan Parameter Sets" class="Arr (strict)"() -> ("Index Values"=w1327:u32[])  [unwired: 2 in, 2 out]
        n993 = Index Array(array=w1327, index=0) -> (element=w1324:u32)
        n994 = local write "Load parameters"(FALSE ("Load parameters")) -> ()
        n995 = Index Array(array="Saved AOD Raster Scan Parameter Sets", index=w1324) -> (element=w1323:T26)
        n996 = Unbundle By Name(w1323) -> ("Scan Range AOD (nm) 2"=w1322:dbl, "Step Size AOD (nm) 2"=w1321:dbl, "Scan Speed AOD (nm/s) 2"=w1320:dbl, "Number of scans (AOD) 2"=w1319:u16)
        n997 = flat-sequence {
          tunnel: w1322 -> [w1330]
          tunnel: w1321 -> [w1329]
          tunnel: w1320 -> [w1328]
          tunnel: w1319 -> [w1331]
          frame #0 {
            n998 = local write "Scan Speed (nm/s)"(w1328) -> ()
            n999 = local write "Scan Range (nm)"(w1330) -> ()
            n1000 = local write "Step Size (nm)"(w1329) -> ()
          }
          frame #1 {
            n1001 = property on="Number of F/B Scans (AOD)" class="DigNum (strict)"("Val(Sgnl)"=w1331) -> ()  [unwired: 2 in, 2 out]
          }
        }
      }
      event "Trap 1 (ON/OFF)", "Trap 2 (ON/OFF)": Value Change {
        n1002 = event-data() -> ()  [unwired: 7 out]
        n1003 = property on="Trap 2 ON" class="Bool (strict)"("Val(Sgnl)"="Trap 2 (ON/OFF)") -> ()  [unwired: 2 in, 2 out]
        n1004 = property on="Trap 1 ON" class="Bool (strict)"("Val(Sgnl)"="Trap 1 (ON/OFF)") -> ()  [unwired: 2 in, 2 out]
      }
      event "DIO count 1 (ticks)", "DIO count 2 (ticks)", "DIO count 3 (ticks)", "Interlace", "Number Interlace Sets", "Not-Interlacing Set": Value Change {
        n1005 = event-data() -> ()  [unwired: 7 out]
        n1006 = local read "DIO count 3 (ticks)"() -> (w1344:u32)
        n1007 = local read "DIO count 1 (ticks)"() -> (w1346:u32)
        n1008 = local read "DIO count 2 (ticks)"() -> (w1345:u32)
        n1009 = To Unsigned Byte Integer(number="Not-Interlacing Set") -> (unsigned 8bit integer=w1335:u8)
        n1010 = Add(x=w1335, y=u8 1) -> (x+y=w1339:u8)
        n1011 = xnode "Read/Write Control"("FPGA VI Reference In"=w1350, "error in"=w1348, "DIO count 1 (ticks)"=w1346, "DIO count 2 (ticks)"=w1345, "DIO count 3 (ticks)"=w1344, "Interlace ON/OFF"="Interlace", "Number Interlace Cycles"="Number Interlace Sets", "Interlace Off Parameters"=w1339) -> ("error out"=w1349:errorcluster)  [unwired: 1 out]
        n1012 = Build Array(w1346, w1345, w1344) -> (w1337:u32[])
        n1013 = Split 1D Array(array=w1337, index="Number Interlace Sets") -> (first subarray=w1347:u32[])  [unwired: 1 out]
        n1014 = Index Array(array=w1337, index=w1335) -> (element=w1336:u32)
        n1015 = Add Array Elements(numeric array=w1347) -> (sum=w1341:u32)
        n1016 = Select(t=w1341, s="Interlace", f=w1336) -> (s? t:f=→"Total Counts (ticks)":u32)
      }
      event "Reset Feedback": Value Change {
        n1017 = event-data() -> ()  [unwired: 7 out]
        n1018 = Unbundle By Name("Reset Feedback") -> ("Set 1"=w1354:bool, "Set 2"=w1353:bool)
        n1019 = xnode "Read/Write Control"("FPGA VI Reference In"=w1356, "error in"=w1351, "FB Reset Set 1"=w1354, "FB Reset Set 2"=w1353) -> ("error out"=w1352:errorcluster)  [unwired: 1 out]
      }
      event "PID Gains": Value Change {
        n1020 = event-data() -> ()  [unwired: 7 out]
        n1021 = Unbundle By Name("PID Gains") -> ("Set 1"=w1360:T14, "Set 2"=w1359:T14)
        n1022 = xnode "Read/Write Control"("FPGA VI Reference In"=w1361, "error in"=w1357, "FB Gains Set 1"=w1360, "FB Gains Set 2"=w1359) -> ("error out"=w1358:errorcluster)  [unwired: 1 out]
      }
      event "AI2 to Setpoint", "Setpoints (V)": Value Change {
        n1023 = event-data() -> ()  [unwired: 7 out]
        n1024 = xnode "Read/Write Control"("FPGA VI Reference In"=w1367, "error in"=w1363) -> ("FPGA VI Reference Out"=w1366:T19, "error out"=w1365:errorcluster, "AI2 Y Sum Set 1"=w1374:i16, "AI2 Y Sum Set 2"=w1373:i16)
        n1025 = Cluster To Array(cluster="AI2 to Setpoint") -> (array=w1377:bool[])
        n1026 = local read "AI2 (V)"() -> (w1375:cluster{"Set 1":dbl, "Set 2":dbl})
        n1027 = Or Array Elements(Boolean array=w1377) -> (logical OR=w1378:bool)
        n1028 = Bundle By Name(cluster=w1375, "Set 1"=w1374, "Set 2"=w1373) -> (w1372:cluster{"Set 1":dbl, "Set 2":dbl})
        n1029 = Divide(x=w1372, y=3276.7) -> (x/y=w1371:cluster{"Set 1":dbl, "Set 2":dbl})
        "AI2 (V)" <- w1371
        n1030 = case shown="True" w1378 {
          tunnel: [w1381 w1398] -> w1370
          tunnel: "AI2 to Setpoint" -> [_ w1394]
          tunnel: "Setpoints (V)" -> [w1382 w1397]
          tunnel: w1371 -> [_ w1391]
          frame False {
            n1031 = Multiply(x=3276.7, y=w1382) -> (x*y=w1383:cluster{"Set 1":dbl, "Set 2":dbl})
            n1032 = To Word Integer(number=w1383) -> (16bit integer=w1381:cluster{"Set 1":i16, "Set 2":i16})
          }
          frame True {
            n1033 = Unbundle By Name(w1391) -> ("Set 1"=w1390:dbl, "Set 2"=w1389:dbl)
            n1034 = Unbundle By Name(w1397) -> ("Set 1"=w1396:dbl, "Set 2"=w1395:dbl)
            n1035 = Unbundle By Name(w1394) -> ("Set 1"=w1393:bool, "Set 2"=w1392:bool)
            n1036 = Select(t=w1390, s=w1393, f=w1396) -> (s? t:f=w1388:dbl)
            n1037 = Select(t=w1389, s=w1392, f=w1395) -> (s? t:f=w1387:dbl)
            n1038 = Bundle By Name(cluster=w1397, "Set 1"=w1388, "Set 2"=w1387) -> (w1385:cluster{"Set 1":dbl, "Set 2":dbl})
            n1039 = local write "Setpoints (V)"(w1385) -> ()
            n1040 = Multiply(x=3276.7, y=w1385) -> (x*y=w1386:cluster{"Set 1":dbl, "Set 2":dbl})
            n1041 = To Word Integer(number=w1386) -> (16bit integer=w1398:cluster{"Set 1":i16, "Set 2":i16})
          }
        }
        n1042 = Unbundle By Name(w1370) -> ("Set 1"=w1369:i16, "Set 2"=w1368:i16)
        n1043 = xnode "Read/Write Control"("FPGA VI Reference In"=w1366, "error in"=w1365, "FB Setpoint Set 1"=w1369, "FB Setpoint Set 2"=w1368) -> ("error out"=w1364:errorcluster)  [unwired: 1 out]
      }
      event "Invert GI": Value Change {
        n1044 = event-data() -> ()  [unwired: 7 out]
        n1045 = xnode "Read/Write Control"("FPGA VI Reference In"=w1403, "error in"=w1401, "Invert GI"="Invert GI", "Invert GI 2"="Invert GI") -> ("error out"=w1402:errorcluster)  [unwired: 1 out]
      }
      event "Green FB Setpoint (mV)", "Green FB Gains", "Green FB On/Off", "Current When FB OFF (%)", "Green int current ON count adj": Value Change {
        n1046 = event-data() -> ()  [unwired: 7 out]
        n1047 = local read "Green FB Setpoint (mV)"() -> (w1410:dbl)
        n1048 = local read "Current When FB OFF (%)"() -> (w1413:dbl)
        n1049 = Multiply(x=w1410, y=3.2767) -> (x*y=w1409:dbl)
        n1050 = Multiply(x=w1413, y=655.35) -> (x*y=w1414:dbl)
        n1051 = To Unsigned Word Integer(number=w1414) -> (unsigned 16bit integer=w1412:u16)
        n1052 = local read "Green int current ON count adj"() -> (w1417:u32)
        n1053 = local read "Green FB Gains"() -> (w1416:T14)
        n1054 = local read "Green Laser ON/Interlacing"() -> (w1407:bool)
        n1055 = local read "Green laser mode"() -> (w1406:enum32{"Laser ON", "Laser OFF", "Interlace"})
        n1056 = local read "Green FB On/Off"() -> (w1418:bool)
        n1057 = Equal?(x=w1406, y=enum32{"Laser ON", "Laser OFF", "Interlace"}."Interlace") -> (x = y?=w1404:bool)
        n1058 = Compound Arithmetic op=AND(w1404, w1418, w1407) -> (w1408:bool)
        n1059 = xnode "Read/Write Control"("FPGA VI Reference In"=w1421, "error in"=w1420, "Green FB Setpoint"=w1409, "Green FB On/Off"=w1408, "Current Out"=w1412, "Green int current ON count adj"=w1417, "Green FB Gains"=w1416) -> ("error out"=w1419:errorcluster)  [unwired: 1 out]
      }
      event "Green laser mode", "Green Laser ON/Interlacing": Value Change {
        n1060 = event-data() -> ()  [unwired: 7 out]
        n1061 = local write "Green Laser ON/OFF"("Green Laser ON/Interlacing") -> ()
        n1062 = case shown="True" "Green Laser ON/Interlacing" {
          tunnel: "Green laser mode" -> [_ w1435]
          tunnel: [enum32{"Laser ON", "Laser OFF", "Interlace"}."Laser OFF" ("Green laser mode") w1435] -> w1424
          tunnel: [FALSE w1431] -> w1423
          frame False {
          }
          frame True {
            n1063 = local read "Green FB On/Off"() -> (w1432:bool)
            n1064 = Equal?(x=w1435, y=enum32{"Laser ON", "Laser OFF", "Interlace"}."Interlace") -> (x = y?=w1433:bool)
            n1065 = And(x=w1433, y=w1432) -> (x .and. y?=w1431:bool)
          }
        }
        n1066 = xnode "Read/Write Control"("FPGA VI Reference In"=w1428, "error in"=w1426, "Operating Mode"=w1424, "Operating Mode 2"=w1424, "Green FB On/Off"=w1423) -> ("error out"=w1427:errorcluster)  [unwired: 1 out]
      }
      event "Green Laser ON/OFF": Value Change {
        n1067 = event-data() -> ()  [unwired: 7 out]
        n1068 = property on="Green Laser ON/Interlacing" class="Bool (strict)"("Val(Sgnl)"="Green Laser ON/OFF") -> ()  [unwired: 2 in, 2 out]
      }
      event "Test ttrig": Value Change {
        n1069 = event-data() -> ()  [unwired: 7 out]
        n1070 = xnode "Read/Write Control"("FPGA VI Reference In"=w1440, "error in"=w1439, "TTrig?"=TRUE) -> ("error out"=w1438:errorcluster)  [unwired: 1 out]
      }
      event "Neg. TTrig FPGA": Value Change {
        n1071 = event-data() -> ()  [unwired: 7 out]
        n1072 = xnode "Read/Write Control"("FPGA VI Reference In"=w1444, "error in"=w1443, "TTrig Negate Pos"="Neg. TTrig FPGA") -> ()  [unwired: 2 out]
      }
      event "- phase (APD 1 Gate)", "+ phase (APD 1 Gate)": Value Change {
        n1073 = event-data() -> ()  [unwired: 7 out]
        n1074 = local read "Phase Adj. (APD 1 Gate)"() -> (w1445:i16)
        n1075 = Negate(x=w1445) -> (-x=w1453:i16)
        n1076 = Select(t=w1453, s="- phase (APD 1 Gate)", f=w1445) -> (s? t:f=w1452:i16)
        n1077 = Or(x="- phase (APD 1 Gate)", y="+ phase (APD 1 Gate)") -> (x .or. y?=w1448:bool)
        n1078 = xnode "Read/Write Control"("FPGA VI Reference In"=w1455, "error in"=w1454, "Phase count adjustment (APD 1 Gate)"=w1452) -> ("FPGA VI Reference Out"=w1450:T19, "error out"=w1451:errorcluster)
        n1079 = xnode "Read/Write Control"("FPGA VI Reference In"=w1450, "error in"=w1451, "+ phase (APD 1 Gate)"=w1448) -> ("error out"=w1449:errorcluster)  [unwired: 1 out]
      }
      event "+ phase (APD 2 Gate)", "- phase (APD 2 Gate)": Value Change {
        n1080 = event-data() -> ()  [unwired: 7 out]
        n1081 = local read "Phase Adj. (APD 2 Gate)"() -> (w1456:i16)
        n1082 = Negate(x=w1456) -> (-x=w1464:i16)
        n1083 = Select(t=w1464, s="- phase (APD 2 Gate)", f=w1456) -> (s? t:f=w1463:i16)
        n1084 = Or(x="- phase (APD 2 Gate)", y="+ phase (APD 2 Gate)") -> (x .or. y?=w1459:bool)
        n1085 = xnode "Read/Write Control"("FPGA VI Reference In"=w1466, "error in"=w1465, "Phase count adjustment (APD 2 Gate)"=w1463) -> ("FPGA VI Reference Out"=w1461:T19, "error out"=w1462:errorcluster)
        n1086 = xnode "Read/Write Control"("FPGA VI Reference In"=w1461, "error in"=w1462, "+ phase (APD 2 Gate)"=w1459) -> ("error out"=w1460:errorcluster)  [unwired: 1 out]
      }
      event "Phase Adj. (APD Acq)", "+ phase (APD Acq)", "- phase (APD Acq)": Value Change {
        n1087 = event-data() -> ()  [unwired: 7 out]
        n1088 = local read "Phase Adj. (APD Acq)"() -> (w1469:i16)
        n1089 = Negate(x=w1469) -> (-x=w1475:i16)
        n1090 = Select(t=w1475, s="+ phase (APD Acq)", f=w1469) -> (s? t:f=w1474:i16)
